vi "Remove Close Atoms on GB.vi"(8 "Grain Boundary Location (A)":dbl, 9 "Edge Duplication Range":dbl=3.0, 10 "Minimally Allowable Distance (A)":dbl=1.5, 11 "Structure":T1={"Structure Name"="Relax2 Subcrystal Expanded to Box+Relax2 Subcrystal Expanded to Box", "Lattice vector a"=[10.1, 0.0, 0.0], "Lattice vector b"=[0.0, 100.1, 0.0], "Lattice vector c"=[0.0, 0.0, 24.72380952380952], "Atoms Array"=[{"Atom Name"="Cd", "Positions (Direct)"=array496x3[1488 elements], "Positions (Cartesian)"=array496x3[1488 elements]}, {"Atom Name"="Te", "Positions (Direct)"=array480x3[1440 elements], "Positions (Cartesian)"=array480x3[1440 elements]}], "# of atoms"=976} {"Atoms Array"."Positions (Cartesian)" format="%#_4f"; "Atoms Array"."Positions (Direct)" format="%#_4f"}) -> (2 "# of Atoms Removed":i32, 3 "Structure with atoms removed":T1={"Structure Name"="Relax2 Subcrystal Expanded to Box+Relax2 Subcrystal Expanded to Box", "Lattice vector a"=[10.1, 0.0, 0.0], "Lattice vector b"=[0.0, 100.1, 0.0], "Lattice vector c"=[0.0, 0.0, 24.72380952380952], "Atoms Array"=[{"Atom Name"="Cd", "Positions (Direct)"=array496x3[1488 elements], "Positions (Cartesian)"=array496x3[1488 elements]}, {"Atom Name"="Te", "Positions (Direct)"=array480x3[1440 elements], "Positions (Cartesian)"=array480x3[1440 elements]}], "# of atoms"=976} {"Atoms Array"."Positions (Cartesian)" format="%#_4f"; "Atoms Array"."Positions (Direct)" format="%#_4f"})   [LabVIEW 2010]
panel:
  out "Array":dbl[][](array[numeric])
  out "Numeric":i32
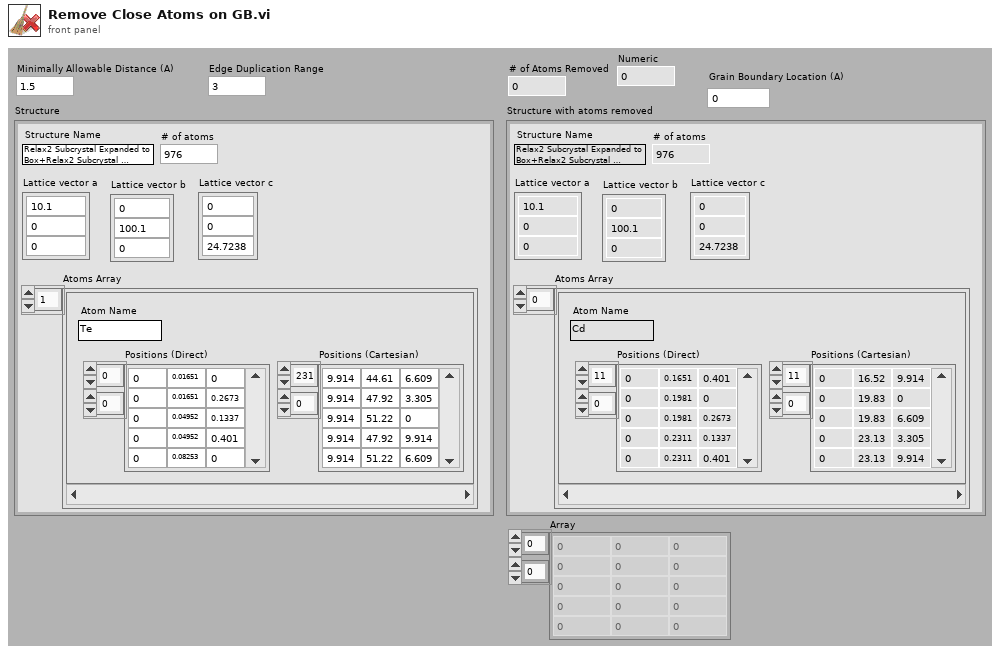
[diagram p1: front panel]
types:
  T1 = cluster{"Structure Name":string, "Lattice vector a":dbl[], "Lattice vector b":dbl[], "Lattice vector c":dbl[], "Atoms Array":cluster{"Atom Name":string, "Positions (Direct)":dbl[][], "Positions (Cartesian)":dbl[][]}[], "# of atoms":i32}
  T2 = cluster{"Atom Name":string, "Positions (Direct)":dbl[][], "Positions (Cartesian)":dbl[][]}[]
  T3 = cluster{"Atom Name":string, "Positions (Direct)":dbl[][], "Positions (Cartesian)":dbl[][]}
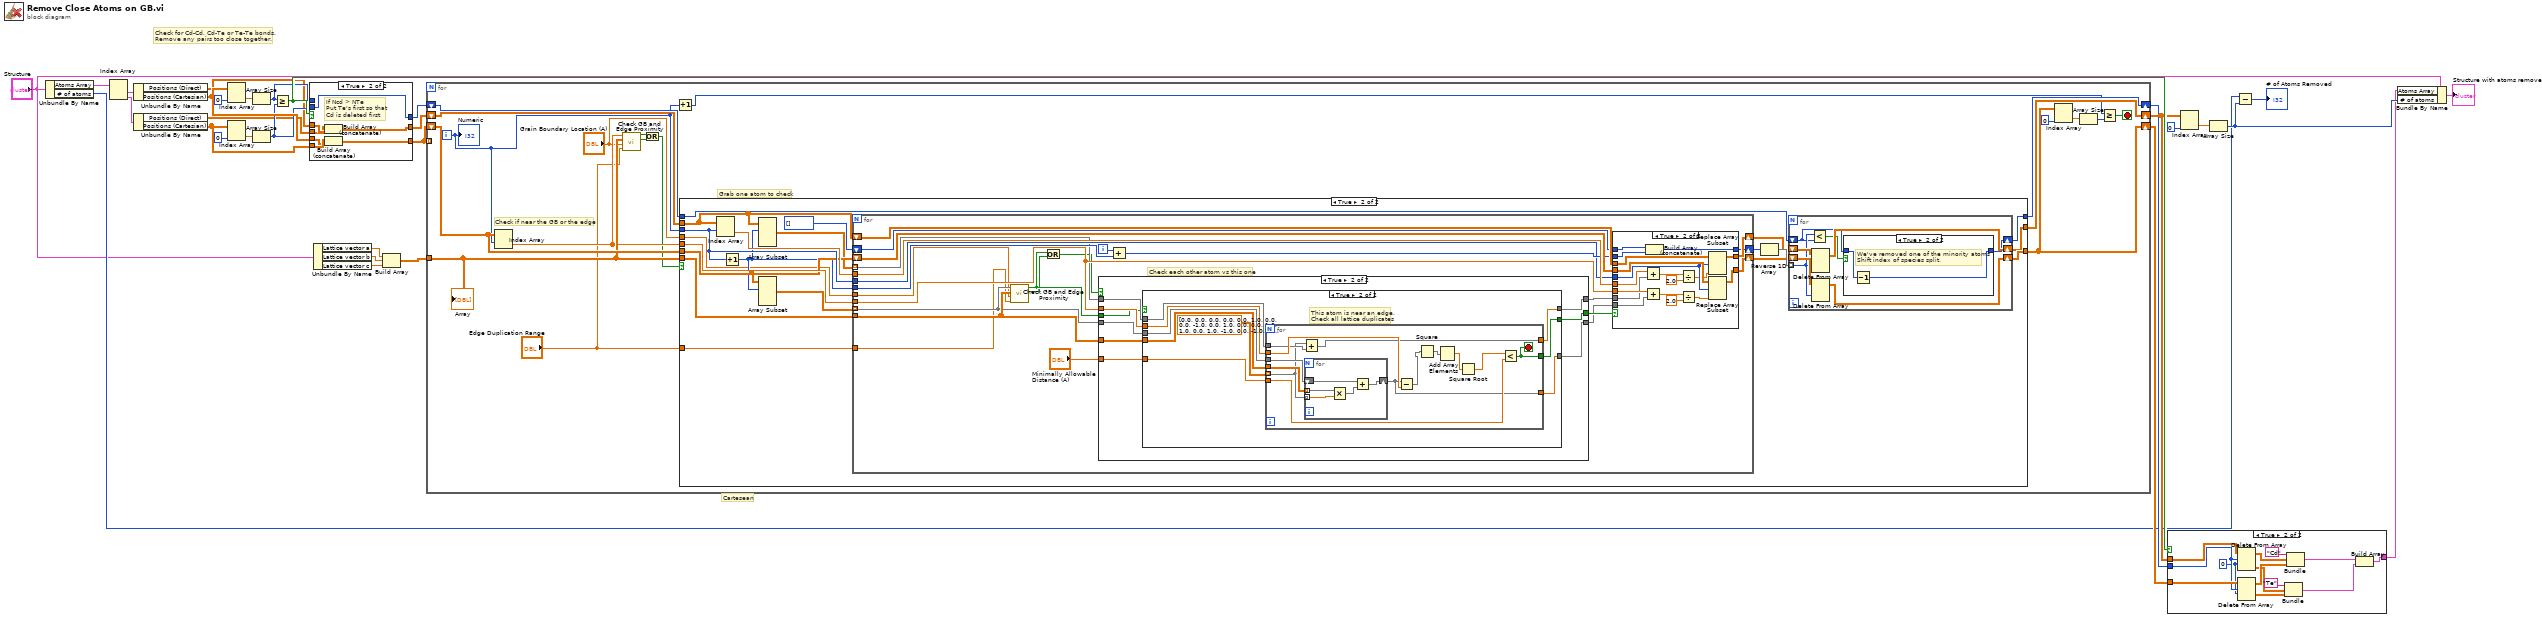
[diagram p0: block diagram]
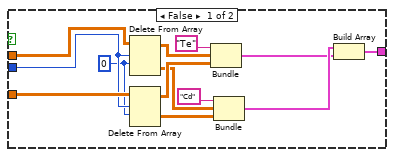
[diagram p2: hidden frame]
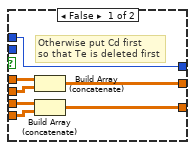
[diagram p3: hidden frame]
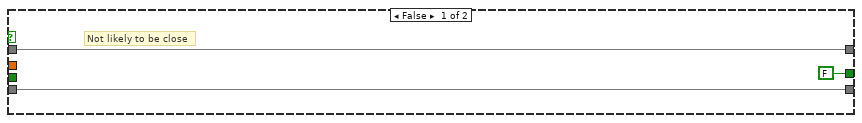
[diagram p5: hidden frame]
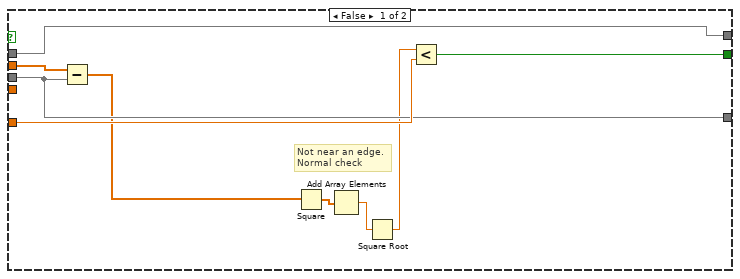
[diagram p6: hidden frame]
diagram:
  # "Cartesean"
  # "Check for Cd-Cd, Cd-Te or Te-Te bonds.\nRemove any pairs too close together."
  n1 = Unbundle By Name("Structure") -> ("Atoms Array"=w31:T2, "# of atoms"=w9:i32)
  n2 = Index Array(array=w31) -> (element #1=w30:T3, element #2=w29:T3)  [unwired: 2 in]
  n3 = Unbundle By Name(w30) -> ("Positions (Direct)"=w16:dbl[][], "Positions (Cartesian)"=w24:dbl[][])
  n4 = Unbundle By Name(w29) -> ("Positions (Direct)"=w15:dbl[][], "Positions (Cartesian)"=w23:dbl[][])
  n5 = Index Array(array=w24, index (col)=0 ("disabled index (col)")) -> (element=w27:dbl[])  [unwired: 1 in]
  n6 = Index Array(array=w23, index (col)=0 ("disabled index (col)")) -> (element=w25:dbl[])  [unwired: 1 in]
  n7 = Array Size(array=w27) -> (size(s)=w19:i32)
  n8 = Array Size(array=w25) -> (size(s)=w20:i32)
  n9 = Greater Or Equal?(x=w19, y=w20) -> (x >= y?=w21:bool)
  n10 = case shown="True" w21 {
    tunnel: w24 -> [w39 w45]
    tunnel: [w38 w44] -> w3
    tunnel: w23 -> [w37 w46]
    tunnel: [w36 w43] -> w18
    tunnel: w20 -> [_ w43]
    tunnel: w19 -> [w36 _]
    tunnel: w16 -> [w35 w42]
    tunnel: w15 -> [w34 w41]
    tunnel: [w33 w40] -> w14
    frame False {
      # "Otherwise put Cd first\nso that Te is deleted first"
      n11 = Build Array (concatenate)(w35, w34) -> (w33:dbl[][])
      n12 = Build Array (concatenate)(w39, w37) -> (w38:dbl[][])
    }
    frame True {
      # "If Ncd > NTe\nPut Te's first so that\nCd is deleted first"
      n13 = Build Array (concatenate)(w41, w42) -> (w40:dbl[][])
      n14 = Build Array (concatenate)(w46, w45) -> (w44:dbl[][])
    }
  }
  n15 = Unbundle By Name("Structure") -> ("Lattice vector a"=w6:dbl[], "Lattice vector b"=w7:dbl[], "Lattice vector c"=w5:dbl[])
  n16 = Build Array(w6, w7, w5) -> (w4:dbl[][])
  n17 = for {
    shift-right: [w60] -> w22
    shift-left: w3 -> [w61]
    shift-right: [w57] -> w17
    shift-left: w18 -> [w58]
    shift-right: [w59] -> w13
    shift-left: w14 -> [w56]
    tunnel: w4 -> [w54]
    tunnel: w3 -> [_] mode=indexing
    i -> [w48]
    stop <- w62 stop-if-true
    # "Grab one atom to check"
    # "Check if near the GB or the edge"
    n18 = Index Array(array=w61, index (row)=w48) -> (element=w53:dbl[])  [unwired: 1 in]
    n19 = call "Check GB and Edge Proximity.vi"("Border Radius"="Edge Duplication Range", "Grain Boundary Location"="Grain Boundary Location (A)", "Lattice Vectors"=w54, "Atom (Cartesian)"=w53) -> ("Along GB?"=w51:bool, "Along Border?"=w52:bool)  [unwired: 6 in]
    n20 = Or(x=w52, y=w51) -> (x .or. y?=w49:bool)
    n21 = Increment(x=w48) -> (x+1=w55:i32)
    n22 = case shown="True" w49 {
      tunnel: w53 -> [_ w87]
      tunnel: w48 -> [_ w85]
      tunnel: w61 -> [w66 w84]
      tunnel: w54 -> [_ w82]
      tunnel: [w66 w81] -> w60
      tunnel: [w67 w80] -> w59
      tunnel: w58 -> [w68 w79]
      tunnel: [w68 w78] -> w57
      tunnel: w56 -> [w67 w77]
      tunnel: "Grain Boundary Location (A)" -> [_ w70]
      tunnel: "Edge Duplication Range" -> [_ w69]
      frame False {
        # "Not likely to be close to another"
      }
      frame True {
        n23 = Index Array(array=w77, index (row)=w85) -> (element=w88:dbl[])  [unwired: 1 in]
        n24 = Increment(x=w85) -> (x+1=w76:i32)
        n25 = Array Subset(array=w77, index (row)=w76) -> (w75:dbl[][])  [unwired: 3 in]
        n26 = Array Subset(array=w84, index (row)=w76) -> (w83:dbl[][])  [unwired: 3 in]
        n27 = for {
          tunnel: w87 -> [w110]
          shift-right: [w112] -> w71
          shift-left: w84 -> [w107]
          tunnel: w85 -> [w97]
          shift-right: [w109] -> w72
          shift-left: w77 -> [w108]
          tunnel: w88 -> [w111]
          shift-right: [w105] -> w74
          shift-left: i32[] [] -> [w104]
          tunnel: w83 -> [w94] mode=indexing
          tunnel: w76 -> [w99]
          tunnel: w82 -> [w95]
          tunnel: w75 -> [w96] mode=indexing
          tunnel: w70 -> [w93]
          tunnel: w69 -> [w89]
          i -> [w100]
          # "Check each other atom vs this one"
          n28 = call "Check GB and Edge Proximity.vi"("Border Radius"=w89, "Grain Boundary Location"=w93, "Lattice Vectors"=w95, "Atom (Cartesian)"=w94) -> ("Along GB?"=w91:bool, "Along Border?"=w92:bool)  [unwired: 6 in]
          n29 = Or(x=w92, y=w91) -> (x .or. y?=w90:bool)
          n30 = case shown="True" w90 {
            tunnel: w110 -> [_ w124]
            tunnel: [FALSE w123] -> w106
            tunnel: "Minimally Allowable Distance (A)" -> [_ w122]
            tunnel: [w114 w121] -> w102
            tunnel: [w115 w120] -> w101
            tunnel: w96 -> [w115 w119]
            tunnel: w95 -> [_ w118]
            tunnel: w94 -> [w114 w117]
            tunnel: w92 -> [_ w116]
            frame False {
              # "Not likely to be close"
            }
            frame True {
              n31 = case shown="True" w116 {
                tunnel: w117 -> [w130 w140]
                tunnel: w122 -> [w132 w139]
                tunnel: w124 -> [w133 w141]
                tunnel: [w131 w138] -> w123
                tunnel: [w130 w135] -> w121
                tunnel: w119 -> [w129 w137]
                tunnel: [w129 w136] -> w120
                tunnel: w118 -> [_ w134]
                frame False {
                  # "Not near an edge.\nNormal check"
                  n32 = Subtract(x=w133, y=w130) -> (x-y=w126:dbl[])
                  n33 = Square(x=w126) -> (x^2=w128:dbl[])
                  n34 = Add Array Elements(numeric array=w128) -> (sum=w127:dbl)
                  n35 = Square Root(x=w127) -> (sqrt(x)=w125:dbl)
                  n36 = Less?(x=w125, y=w132) -> (x < y?=w131:bool)
                }
                frame True {
                  # "This atom is near an edge.\nCheck all lattice duplicates"
                  n37 = for {
                    tunnel: w140 -> [w155]
                    tunnel: dbl[][] [[0.0, 0.0, 0.0], [0.0, 0.0, 1.0], [0.0, 0.0, -1.0], [0.0, 1.0, 0.0], [0.0, 1.0, 1.0], [0.0, 1.0, -1.0], [0.0, -1.0, 0.0], [0.0, -1.0, 1.0], [0.0, -1.0, -1.0], [1.0, 0.0, 0.0], [1.0, 0.0, 1.0], [1.0, 0.0, -1.0], [1.0, 1.0, 0.0], [1.0, 1.0, 1.0], [1.0, 1.0, -1.0], [1.0, -1.0, 0.0], [1.0, -1.0, 1.0], [1.0, -1.0, -1.0], [-1.0, 0.0, 0.0], [-1.0, 0.0, 1.0], [-1.0, 0.0, -1.0], [-1.0, 1.0, 0.0], [-1.0, 1.0, 1.0], [-1.0, 1.0, -1.0], [-1.0, -1.0, 0.0], [-1.0, -1.0, 1.0], [-1.0, -1.0, -1.0]] ("Array") -> [w147] mode=indexing
                    tunnel: [w148] -> w135
                    tunnel: w134 -> [w154]
                    tunnel: w141 -> [w153]
                    tunnel: w139 -> [w152]
                    tunnel: [w151] -> w138
                    tunnel: [w150] -> w136
                    tunnel: w137 -> [w149]
                    stop <- w151 stop-if-true
                    n38 = Add(x=w147, y=w149) -> (x+y=w150:dbl[])
                    n39 = for {
                      shift-right: [w156] -> w148
                      shift-left: w155 -> [w157]
                      tunnel: w147 -> [w160] mode=indexing
                      tunnel: w154 -> [w159] mode=indexing
                      n40 = Multiply(x=w159, y=w160) -> (x*y=w158:dbl[])
                      n41 = Add(x=w157, y=w158) -> (x+y=w156:dbl[])
                    }
                    n42 = Subtract(x=w148, y=w153) -> (x-y=w144:dbl[])
                    n43 = Square(x=w144) -> (x^2=w146:dbl[])
                    n44 = Add Array Elements(numeric array=w146) -> (sum=w145:dbl)
                    n45 = Square Root(x=w145) -> (sqrt(x)=w143:dbl)
                    n46 = Less?(x=w143, y=w152) -> (x < y?=w151:bool)
                  }
                }
              }
            }
          }
          n47 = Add(x=w100, y=w99) -> (x+y=w98:i32)
          n48 = case shown="True" w106 {
            tunnel: w107 -> [w163 w177]
            tunnel: [w163 w167] -> w112
            tunnel: w97 -> [_ w173]
            tunnel: w102 -> [_ w179]
            tunnel: w110 -> [_ w178]
            tunnel: w108 -> [w162 w174]
            tunnel: [w162 w168] -> w109
            tunnel: w101 -> [_ w171]
            tunnel: w111 -> [_ w170]
            tunnel: [w161 w166] -> w105
            tunnel: w104 -> [w161 w165]
            tunnel: w98 -> [_ w164]
            frame False {
            }
            frame True {
              n49 = Add(x=w170, y=w171) -> (x+y=w172:dbl[])
              n50 = Add(x=w178, y=w179) -> (x+y=w180:dbl[])
              n51 = Build Array (concatenate)(w165, w164) -> (w166:i32[])
              n52 = Divide(x=w172, y=2.0) -> (x/y=w169:dbl[])
              n53 = Divide(x=w180, y=2.0) -> (x/y=w176:dbl[])
              n54 = Replace Array Subset(array=w174, new element=w169, index (row)=w173) -> (w168:dbl[][])  [unwired: 1 in]
              n55 = Replace Array Subset(array=w177, new element=w176, index (row)=w173) -> (w167:dbl[][])  [unwired: 1 in]
            }
          }
        }
        n56 = Reverse 1D Array(array=w74) -> (reversed array=w73:i32[])
        n57 = for {
          shift-right: [w188] -> w80
          shift-left: w72 -> [w189]
          tunnel: w73 -> [w184] mode=indexing
          shift-right: [w186] -> w81
          shift-left: w71 -> [w187]
          shift-right: [w185] -> w78
          shift-left: w79 -> [w183]
          n58 = Less?(x=w184, y=w183) -> (x < y?=w182:bool)
          n59 = Delete From Array(array=w189, index (row)=w184) -> (array with subset deleted=w188:dbl[][])  [unwired: 2 in, 1 out]
          n60 = Delete From Array(array=w187, index (row)=w184) -> (array with subset deleted=w186:dbl[][])  [unwired: 2 in, 1 out]
          n61 = case shown="True" w182 {
            tunnel: [w190 w192] -> w185
            tunnel: w183 -> [w190 w191]
            frame False {
            }
            frame True {
              # "We've removed one of the minority atoms\nShift index of species split."
              n62 = Decrement(x=w191) -> (x-1=w192:i32)
            }
          }
        }
      }
    }
    n63 = Index Array(array=w60, index (col)=0 ("disabled index (col)")) -> (element=w64:dbl[])  [unwired: 1 in]
    n64 = Array Size(array=w64) -> (size(s)=w63:i32)
    n65 = Greater Or Equal?(x=w55, y=w63) -> (x >= y?=w62:bool)
    "Numeric" <- w48
    "Array" <- w54
  }
  n66 = case shown="True" w21 {
    tunnel: w22 -> [w205 w218]
    tunnel: [w200 w215] -> w2
    tunnel: w17 -> [w196 w209]
    tunnel: w13 -> [w197 w210]
    frame False {
      w195 = 0 ("index (row)")
      n67 = Delete From Array(array=w197, length=w196, index (row)=w195) -> (deleted portion=w194:dbl[][], array with subset deleted=w193:dbl[][])  [unwired: 1 in]
      n68 = Delete From Array(array=w205, length=w196, index (row)=w195) -> (deleted portion=w199:dbl[][], array with subset deleted=w198:dbl[][])  [unwired: 1 in]
      n69 = Bundle("Te", w193, w198) -> (w201:cluster{string, dbl[][], dbl[][]})  [unwired: 1 in]
      n70 = Bundle("Cd", w194, w199) -> (w203:cluster{string, dbl[][], dbl[][]})  [unwired: 1 in]
      n71 = Build Array(w203, w201) -> (w200:cluster{string, dbl[][], dbl[][]}[])
    }
    frame True {
      w208 = 0 ("index (row)")
      n72 = Delete From Array(array=w210, length=w209, index (row)=w208) -> (deleted portion=w206:dbl[][], array with subset deleted=w207:dbl[][])  [unwired: 1 in]
      n73 = Delete From Array(array=w218, length=w209, index (row)=w208) -> (deleted portion=w212:dbl[][], array with subset deleted=w211:dbl[][])  [unwired: 1 in]
      n74 = Bundle("Te", w206, w212) -> (w213:cluster{string, dbl[][], dbl[][]})  [unwired: 1 in]
      n75 = Bundle("Cd", w207, w211) -> (w216:cluster{string, dbl[][], dbl[][]})  [unwired: 1 in]
      n76 = Build Array(w216, w213) -> (w215:cluster{string, dbl[][], dbl[][]}[])
    }
  }
  n77 = Index Array(array=w13, index (col)=0 ("disabled index (col)")) -> (element=w11:dbl[])  [unwired: 1 in]
  n78 = Array Size(array=w11) -> (size(s)=w10:i32)
  n79 = Subtract(x=w9, y=w10) -> (x-y=→"# of Atoms Removed":i32)
  n80 = Bundle By Name(cluster="Structure", "Atoms Array"=w2, "# of atoms"=w10) -> (→"Structure with atoms removed":T1)
